vi "Добавить точку на рисунок (SubVI).vi"(0 "in picture":picture, 1 "dot х":u16 step=1, 2 "dot y":u16 step=1, 3 "thickness":u16 step=1, 4 "цвет":u32(colorbox), 5 "error in":errorcluster) -> (10 "Коорд.X":u16 step=1, 11 "Коорд.Y":u16 step=1, 14 "error out":errorcluster, 19 "out picture":picture)   [LabVIEW 2013]
panel:
  in  "Style":T1(ring)
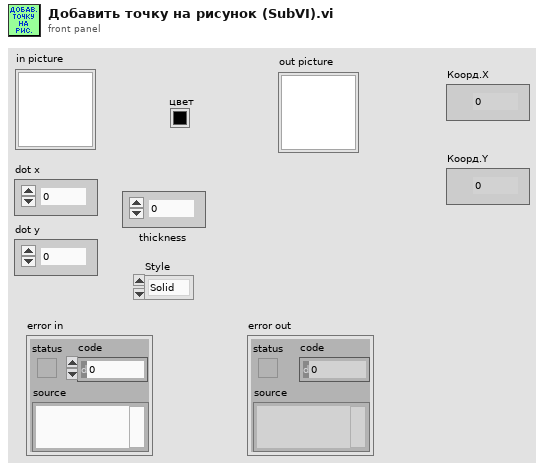
[diagram p1: front panel]
types:
  T1 = enum32{"Solid", "Dash", "Dot", "DashDot", "DashDotDot"}
  T2 = cluster{"thickness":u16, "Style":enum32{"Solid", "Dash", "Dot", "DashDot", "DashDotDot"}}
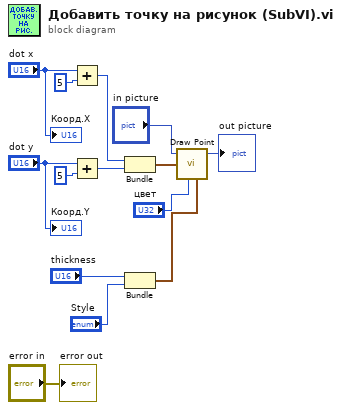
[diagram p0: block diagram]
diagram:
  n1 = Add(x="dot х", y=u16 5) -> (x+y=w3:u16)
  n2 = Add(x="dot y", y=u16 5) -> (x+y=w4:u16)
  n3 = Bundle(w3, w4) -> (w10:cluster{u16, u16})  [unwired: 1 in]
  n4 = Bundle("thickness"="thickness", "Style"="Style") -> (w13:T2)  [unwired: 1 in]
  n5 = call <vilib>:"Draw Point.vi"("picture"="in picture", "point(x,y)"=w10, "color(black)"="цвет", "pen"=w13) -> ("new picture"=→"out picture":picture)  [unwired: 5 in]
  "error out" <- "error in"
  "Коорд.X" <- "dot х"
  "Коорд.Y" <- "dot y"
